vi "Do.vi"(8 "error in (no error)":errorcluster, 10 "Actor in":refnum<class "Actor.lvclass">, 11 "Write StationOptions Msg":refnum<class "Write StationOptions Msg.lvclass">) -> (0 "error out":errorcluster, 2 "Actor out":refnum<class "Actor.lvclass">)   [LabVIEW 2019, in "TestBench.lvlib" / "Write StationOptions Msg.lvclass"]
doc: "This VI delivers the message to the actor by calling the appropriate method(s) on the actor."
uses:
  Write StationOptions Msg.lvclass
  C:/Program Files (x86)/National Instruments/LabVIEW 2019/vi.lib/NI/Event Source Actor/Event Source/Event Source Messages/Event Generated Msg/Event Generated Msg.lvclass
  <vilib>/ActorFramework/Actor/Actor.lvclass
  TestBench/TestBench.lvclass
  C:/Program Files (x86)/National Instruments/LabVIEW 2019/vi.lib/ActorFramework/Actor/Actor.lvclass
  SoftwareSetup/SoftwareSetup/StationOptions.lvclass
  <vilib>/NI/Event Source Actor/Event Source/Event Source Messages/Event Generated Msg/Event Generated Msg.lvclass/Event Generated Msg.ctl
  <vilib>/NI/Event Source Actor/Event Source/Event Source Messages/Event Generated Msg/Event Generated Msg.lvclass
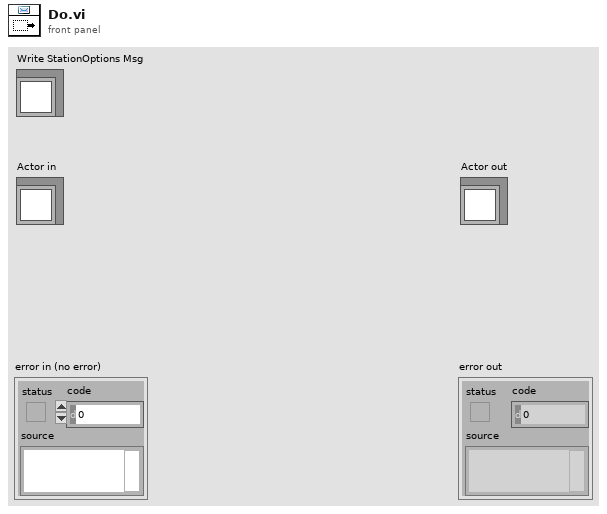
[diagram p1: front panel]
types:
  T1 = typedef "SoftwareSetup.lvlib/DataBase.ctl" = cluster{"Connection String Expression":string, "User ID":string, "Password":string}
  T2 = typedef "SoftwareSetup.lvlib/Local Report.ctl" = cluster{"Report Path":path, "Report  Format":enum16{"CSV", "XML", "PDF", "Excel", "TXT"}, "Disabled State":bool, "Customer name":string}
  T3 = typedef "SoftwareSetup.lvlib/Localization.ctl" = cluster{"Language":enum16{"English", "Chinese"}}
  T4 = typedef "SoftwareSetup.lvlib/Preferences.ctl" = cluster{"Station ID":string, "IP Address":string, "Password":string}
  T5 = typedef "SoftwareSetup.lvlib/User Manager.ctl" = cluster{"Current User Manager File":string, "Login on start":bool}
  T6 = typedef "SoftwareSetup.lvlib/Multiple UUT Settings.ctl" = cluster{"Number of Tests Sockets":u8, "Synchronization":enum16{"Don't Synchronize", "Serial", "Parallel", "One Thread Only"}}
  T7 = typedef "SoftwareSetup.lvlib/Sequence.ctl" = cluster{"Sequence Folder Path":path}
  T8 = cluster{"DataBase":T1, "Local Report":T2, "Localization":T3, "Preferences":T4, "  User Manager":T5, "Multiple UUT Settings":T6, "Sequence":T7}
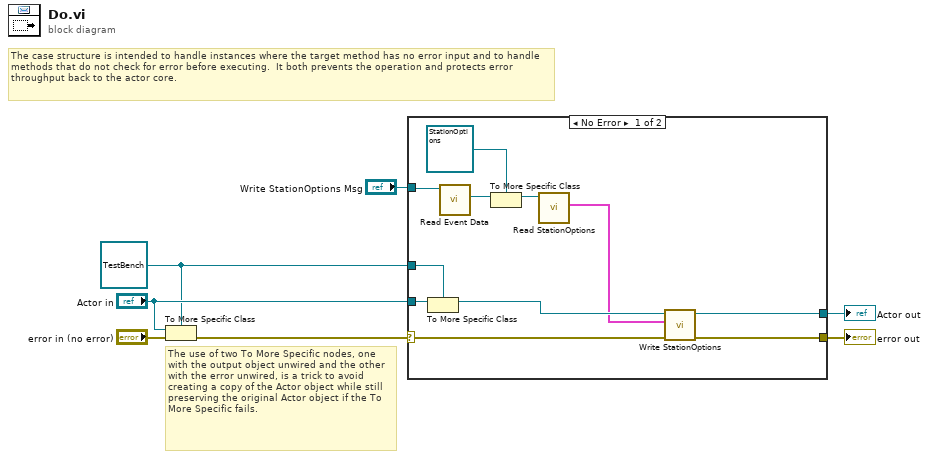
[diagram p0: block diagram]
diagram:
  w2 = refnum<class "TestBench.lvclass"> refnum ("Actor in")
  # "The use of two To More Specific nodes, one with the output object unwired and the other with the error unwired, is a trick to avoid creating a copy of the Actor object while still preserving the original Actor object if the To More Specific fails."
  # "The case structure is intended to handle instances where the target method has no error input and to handle methods that do not check for error before executing.  It both prevents the operation and protects error throughput back to the actor core."
  n1 = To More Specific Class(target class=w2, reference="Actor in", error in="error in (no error)") -> (error out=w6:errorcluster)  [unwired: 1 out]
  n2 = case shown="No Error" w6 {
    selector: w6 -> [w16 w20]
    tunnel: [w18 w20] -> w5
    tunnel: [w17 w19] -> w4
    tunnel: "Actor in" -> [w15 w19]
    tunnel: w2 -> [w14 _]
    tunnel: "Write StationOptions Msg" -> [w12 _]
    frame No Error {
      n3 = To More Specific Class(target class=w14, reference=w15) -> (specific class reference=w13:refnum<class "TestBench.lvclass">)  [unwired: 1 in, 1 out]
      n4 = call <vilib>:"Read Event Data.vi"("Event Generated Msg"=w12) -> ("Event Data"=w11:refnum<class "Event.lvclass">)  [unwired: 10 in]
      n5 = To More Specific Class(target class=refnum<class "StationOptions.lvclass"> refnum ("SoftwareSetup.lvlib:StationOptions.lvclass"), reference=w11) -> (specific class reference=w9:refnum<class "StationOptions.lvclass">)  [unwired: 1 in, 1 out]
      n6 = call-dynamic "Read StationOptions.vi"("StationOptions in"=w9) -> ("StationOptions"=w8:T8)  [unwired: 8 in, 2 out]
      n7 = call-dynamic "Write StationOptions.vi"("error in (no error)"=w16, "StationOptions"=w8, "TestBench in"=w13) -> ("error out"=w18:errorcluster, "TestBench out"=w17:refnum<class "TestBench.lvclass">)  [unwired: 7 in]
    }
    frame Error {
      # "If type check fails, pass the original object out again."
    }
  }
  "error out" <- w5
  "Actor out" <- w4
